vi "Two Buttons Dialog Window with Resizeable Message.vi"(0 "Message":string, 1 "Return =  OK (T)":bool=TRUE, 2 "OK Button Text":string="OK", 3 "Cancel Button Text":string="Cancel", 4 "ESC =  Cancel (T)":bool=TRUE) -> (7 "OK?":bool)   [LabVIEW 2021, in "GUI.lvlib"]
uses:
  GUI.lvlib
  <vilib>/Utility/miscctls.llb/LVKeyTypeDef.ctl
  Error/Error.lvlib
panel:
  in  "Checkbox":bool
  in  "Cancel":bool
  in  "OK":bool
  out "Displayed Message":string
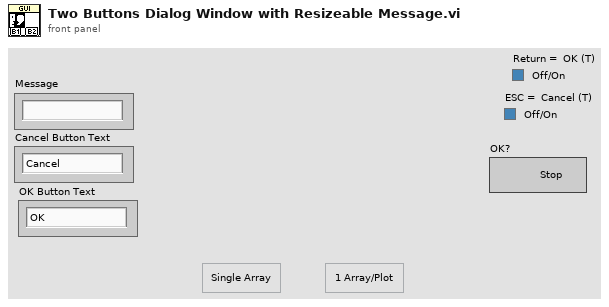
[diagram p1: front panel]
types:
  T1 = typedef "LVKeyTypeDef.ctl" = cluster{"Focus":bool, "Control":bool, "Shift":bool, "Key":string}
  T2 = cluster{"Displayed Message":refnum<vi>, "Checkbox":refnum<vi>, "Cancel":refnum<vi>, "OK":refnum<vi>}
  T3 = enum32{"Invalid", "Standard", "Closed", "Hidden", "Minimized", "Maximized"}
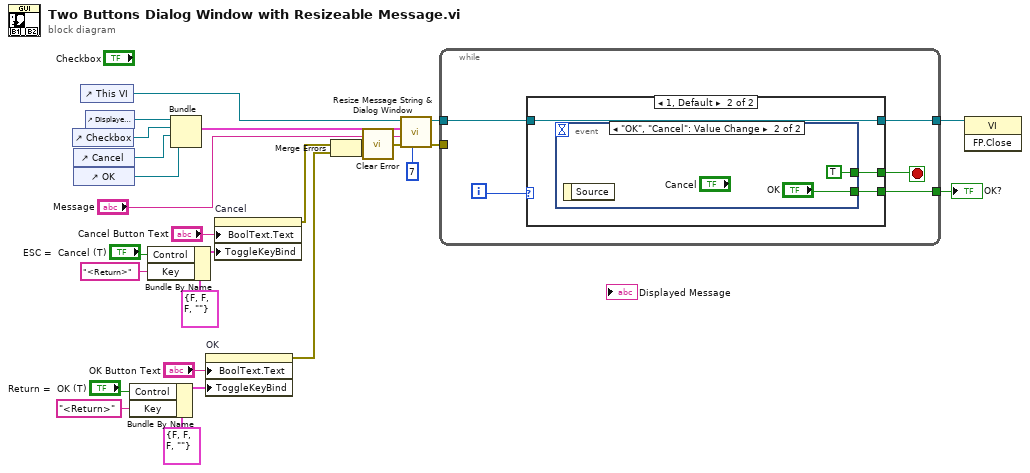
[diagram p0: block diagram]
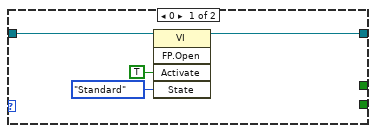
[diagram p2: hidden frame]
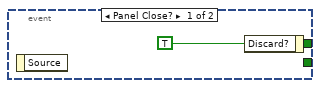
[diagram p3: hidden frame]
diagram:
  n1 = control-ref of="Checkbox"() -> (w14:refnum<vi>)
  n2 = control-ref of="Cancel"() -> (w15:refnum<vi>)
  n3 = control-ref of="OK"() -> (w21:refnum<vi>)
  n4 = control-ref of="This VI"() -> (w20:refnum<vi>)
  n5 = control-ref of="Displayed Message"() -> (w22:refnum<vi>)
  n6 = Bundle By Name(cluster=T1 {"Focus"=FALSE, "Control"=FALSE, "Shift"=FALSE, "Key"=""} ("Toggle Key Binding"), "Control"="Return =  OK (T)", "Key"="<Return>") -> (w3:T1)
  n7 = Bundle By Name(cluster=T1 {"Focus"=FALSE, "Control"=FALSE, "Shift"=FALSE, "Key"=""} ("Toggle Key Binding"), "Control"="ESC =  Cancel (T)", "Key"="<Return>") -> (w8:T1)
  n8 = Bundle("Displayed Message"=w22, "Checkbox"=w14, "Cancel"=w15, "OK"=w21) -> (w19:T2)  [unwired: 1 in]
  n9 = property on="OK" class="Bool"("BoolText.Text"="OK Button Text", "ToggleKeyBind"=w3) -> (error out=w11:errorcluster)  [unwired: 2 in, 1 out]
  n10 = property on="Cancel" class="Bool"("BoolText.Text"="Cancel Button Text", "ToggleKeyBind"=w8) -> (error out=w13:errorcluster)  [unwired: 2 in, 1 out]
  n11 = Merge Errors(w13, w11) -> (w12:errorcluster)
  n12 = call "Clear Error.vi"("Error In"=w12) -> ("no Error Out"=w1:errorcluster)  [unwired: 8 in]
  n13 = call "Resize Message String & Dialog Window.vi"("Max Number of Lines"=7, "Error In"=w1, "Message"="Message", "Controls & Indicators"=w19, "VI Refnum"=w20) -> ("Error Out"=w10:errorcluster, "VI Refnum out"=w16:refnum<vi>)  [unwired: 5 in]
  n14 = while {
    tunnel: w16 -> [w28]
    tunnel: [w27] -> w26
    tunnel: [w30] -> w23
    tunnel: w10 -> [_]
    i -> [w29]
    stop <- w31 stop-if-true
    n15 = case shown="1, Default" w29 {
      tunnel: [_ w38] -> w31
      tunnel: [_ w37] -> w30
      tunnel: w28 -> [w35 w36]
      tunnel: [w34 w36] -> w27
      frame 0 {
        n16 = invoke class="VI" method="FP.Open"(reference=w35, "Activate"=TRUE ("Activate?"), "State"=T3."Standard") -> (reference out=w34:refnum<vi>)  [unwired: 2 in, 4 out]
      }
      frame 1, Default {
        n17 = event shown="[1] \"OK\", \"Cancel\": Value Change" {
          selector: _ -> [_ _]
          dyn-events: _ -> [_ _]
          timeout: _ -> [_ _]
          tunnel: [w39 TRUE ("Discard?")] -> w38
          tunnel: [_ "OK"] -> w37
          event Panel Close? {
            w39 = TRUE ("Discard?")
            n18 = event-data() -> ()  [unwired: 1 in, 1 out]
            n19 = event-data("Discard?"=w39) -> ()  [unwired: 1 in, 1 out]
          }
          event "OK", "Cancel": Value Change {
            n20 = event-data() -> ()  [unwired: 1 in, 1 out]
          }
        }
      }
    }
  }
  "OK?" <- w23
  n21 = invoke class="VI" method="FP.Close"(reference=w26) -> ()  [unwired: 2 in, 3 out]
